vi "Add Response_ex1.vi"() -> ()   [LabVIEW 2019]
uses:
  <vilib>/NI VeriStand/Custom Device API/Custom Device Item Ref.ctl
  Control 7.ctl
  Scripting API/Polymorphic/Add Response_Byte count.vi
  Scripting API/Scripting API.lvlib
  <vilib>/NI VeriStand/Custom Device API/Custom Device API.lvlib
panel:
  out "response refnum":T1=18446744073709551615 format="%.0x"
  out "message refnum out":T1=18446744073709551615 format="%.0x"
  out "error out":errorcluster
  in  "message refnum in":T1=18446744073709551615 format="%.0x"
  in  "error in (no error)":errorcluster
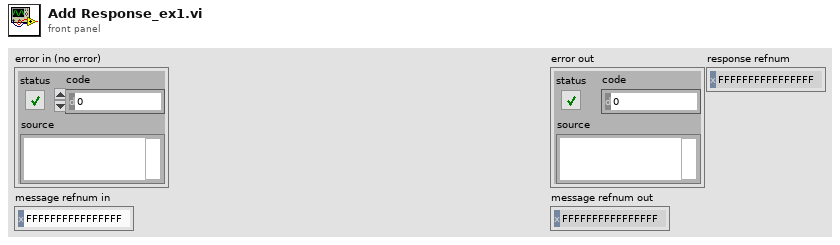
[diagram p1: front panel]
types:
  T1 = typedef "Custom Device API.lvlib/Custom Device Item Ref.ctl" = u64
  T2 = typedef "Control 7.ctl" = cluster{"Response Format":string, "Linkages":cluster{"Variable name":string, "Linked Channel refnum":T1}[], "Byte Count value":u32, "Use Byte Count Channel?":bool, "Channel Refnum":T1}
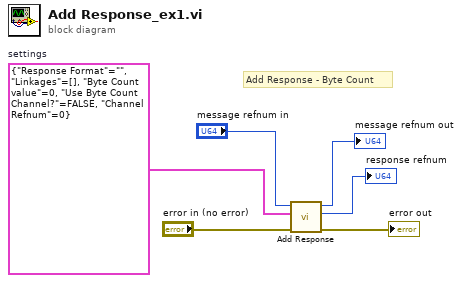
[diagram p0: block diagram]
diagram:
  w2 = T2 {"Response Format"="", "Linkages"=[], "Byte Count value"=0, "Use Byte Count Channel?"=FALSE, "Channel Refnum"=0}  # settings
  # "Add Response - Byte Count"
  n1 = call-poly "Add Response.vi"("Error In"="error in (no error)", "Settings"=w2, "Message Refnum In"="message refnum in") -> ("Error Out"=→"error out":errorcluster, "Response Refnum"=→"response refnum":T1, "Message Refnum Out"=→"message refnum out":T1)  [unwired: 6 in]
